vi "ToString.vi"(8 "error in (no error)":errorcluster, 11 "Theory in":refnum<class "Theory.lvclass">) -> (0 "error out":errorcluster, 2 "String":string, 3 "Theory out":refnum<class "Theory.lvclass">)   [LabVIEW 2017, in "Theory.lvclass"]
doc: "Returns the string representation for this object."
uses:
  Theory.lvclass
  Theory.lvclass/Theory.ctl
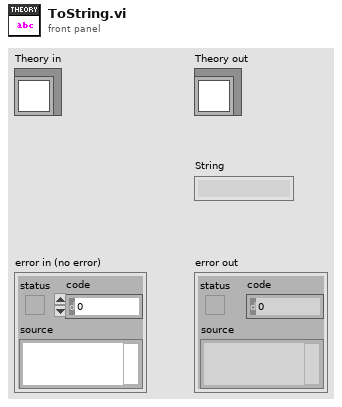
[diagram p1: front panel]
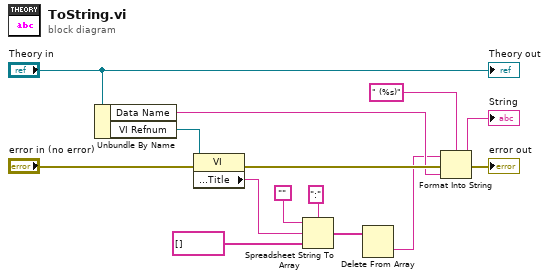
[diagram p0: block diagram]
diagram:
  n1 = Unbundle By Name("Theory in") -> ("Data Name"=w9:string, "VI Refnum"=w11:refnum<vi>)
  n2 = property class="VI"(reference=w11, error in="error in (no error)") -> (error out=w13:errorcluster, "Front Panel.Title"=w1:string)  [unwired: 1 out]
  n3 = Spreadsheet String To Array(delimiter (Tab)=":" ("delimiter"), format string="", spreadsheet string=w1, array type (2D Dbl)=string[] []) -> (array=w2:string[])
  n4 = Delete From Array(array=w2) -> (deleted portion=w6:string)  [unwired: 2 in, 1 out]
  n5 = Format Into String(format string=" (%s)", initial string=w6, error in=w13, w9) -> (resulting string=→"String":string, error out=→"error out":errorcluster)
  "Theory out" <- "Theory in"
